vi "MSG Error.vi"(8 "error in":errorcluster, 9 "Encountered error in":errorcluster, 10 "Sender Name":string) -> (0 "error out":errorcluster)   [LabVIEW 2020, in "GUI.lvlib"]
uses:
  GUI.lvlib
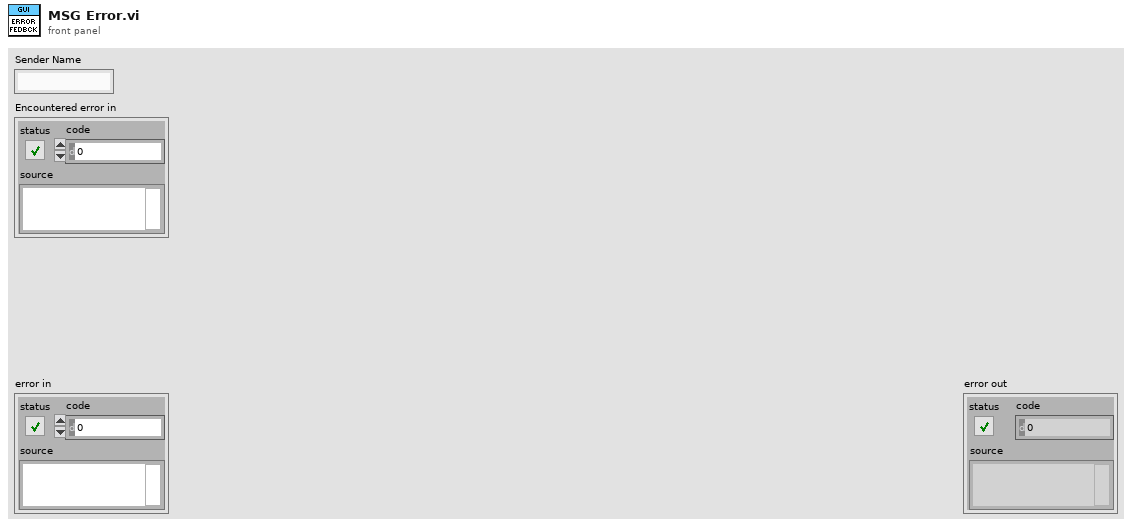
[diagram p1: front panel]
types:
  T1 = cluster{"Sender Name":string, "Encountered error in":errorcluster}
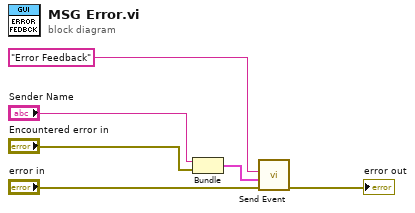
[diagram p0: block diagram]
diagram:
  n1 = Bundle("Sender Name"="Sender Name", "Encountered error in"="Encountered error in") -> (w1:T1)  [unwired: 1 in]
  n2 = call "Send Event.vi"("error in"="error in", "Payload"=w1, "Command"="Error Feedback") -> ("error out"=→"error out":errorcluster)  [unwired: 8 in]
